vi "sensor cmd calibration version.vi"(10 "calibration_version":u32, 11 "device_handle":u32) -> (1 "function return":i32, 2 "calibration_version out":u32, 3 "device_handle out":u32)   [LabVIEW 2019, in "apdm.lvlib"]
doc: "APDM_EXPORT int apdm_sensor_cmd_calibration_version(apdm_device_handle_t device_handle, uint32_t *calibration_version);"
uses:
  apdm.lvlib
  Lee Lab/CP FES Walking 2018/Code/Working/LabVIEW/apdm.dll
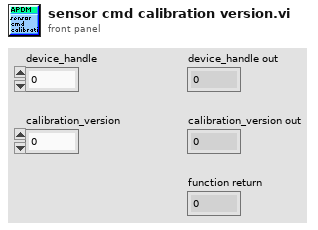
[diagram p1: front panel]
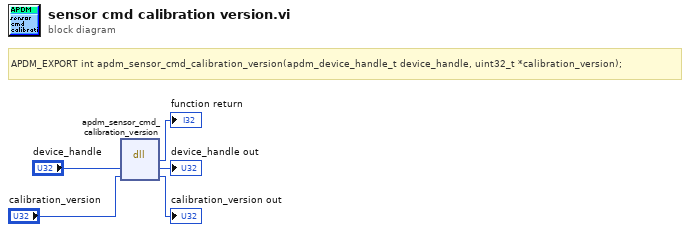
[diagram p0: block diagram]
diagram:
  # "APDM_EXPORT int apdm_sensor_cmd_calibration_version(apdm_device_handle_t device_handle, uint32_t *calibration_version);"
  n1 = dll-call lib="C:/Users/jfalesi/Dropbox/Lee Lab/CP FES Walking 2018/Code/Working/LabVIEW/apdm.*" fn="apdm_sensor_cmd_calibration_version"("device_handle"="device_handle", "calibration_version"="calibration_version") -> (→"function return":i32, "device_handle"=→"device_handle out":u32, "calibration_version"=→"calibration_version out":u32)  [unwired: 3 in, 2 out]
